vi "OpenInstrument.vi"() -> (0 "错误输出":errorcluster, 2 "仪器存在":bool, 3 "VISA资源名称输出":refnum<visa-resource-name>)   [LabVIEW 2020]
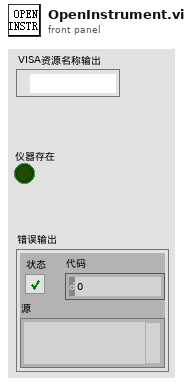
[diagram p1: front panel]
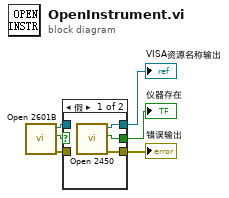
[diagram p0: block diagram]
diagram:
  n1 = call "Open 2601B.vi"() -> ("错误输出"=w3:errorcluster, "仪器存在"=w6:bool, "VISA资源名称输出"=w5:refnum<visa-resource-name>)  [unwired: 9 in]
  n2 = case shown="假" w6 {
    selector: w6 -> [_ w10]
    tunnel: [w9 w12] -> w4
    tunnel: w5 -> [_ w12]
    tunnel: w3 -> [_ w11]
    tunnel: [w8 w11] -> w2
    tunnel: [w7 w10] -> w1
    frame False {
      n3 = call "Open 2450.vi"() -> ("错误输出"=w8:errorcluster, "仪器存在"=w7:bool, "VISA资源名称输出"=w9:refnum<visa-resource-name>)  [unwired: 9 in]
    }
    frame True {
    }
  }
  "VISA资源名称输出" <- w4
  "错误输出" <- w2
  "仪器存在" <- w1
